vi "OpenAllNodes.vi"(0 "Task":T1(ring)) -> (2 "Nodes":cluster{"node":string, "Node Port":i32}[](array[cluster]))   [LabVIEW 2012]
uses:
  SubVIs/_ROSControl.ctl
  SubVIs/_ROSDirection.ctl
  _ROSDefinition.vi
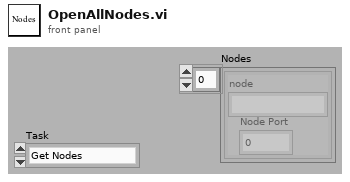
[diagram p1: front panel]
types:
  T1 = enum16{"Get Nodes", "Start Nodes", "Reset Nodes"}
  T2 = typedef "_ROSControl.ctl" = cluster{"topic port":u16, "Node":string, "topic":string, "type":string, "node port":u32, "error ":errorcluster, "Direction":T3, "APIs":string[], "Update (ms)":u16, "write queue":u16}
  T3 = typedef "_ROSDirection.ctl" = enum16{"Node", "Publisher", "Subscriber", "Service Client"}
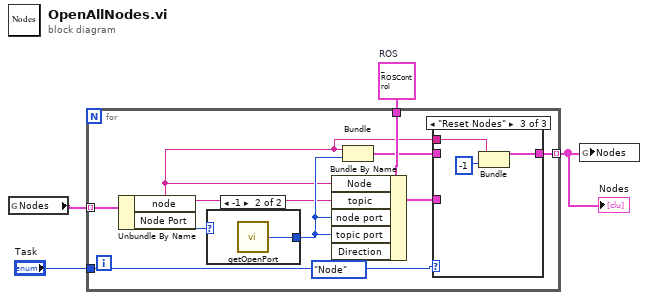
[diagram p0: block diagram]
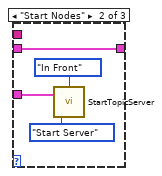
[diagram p3: hidden frame]
diagram:
  w4 = T2 {"topic port"=0, "Node"="", "topic"="", "type"="", "node port"=0, "error "={"status"=FALSE, "code"=0, "source"=""}, "Direction"=enum."Node", "APIs"=[], "Update (ms)"=0, "write queue"=0}  # ROS
  n1 = global read "_ROSDefinition.vi" "Nodes"() -> (w2:cluster{"node":string, "Node Port":i32}[])
  n2 = for {
    tunnel: w2 -> [w14] mode=indexing
    tunnel: w4 -> [w13]
    tunnel: [w6] -> w3 mode=indexing
    tunnel: "Task" -> [w8]
    n3 = Unbundle By Name(w14) -> ("node"=w7:string, "Node Port"=w10:i32)
    n4 = case shown="-1" w10 {
      selector: w10 -> [w23 _]
      tunnel: [w23 w24] -> w9
      frame Default {
      }
      frame -1 {
        n5 = call "getOpenPort.vi"() -> ("port"=w24:u16)
      }
    }
    n6 = Bundle By Name(cluster=w13, "Node"=w7, "topic"=w7, "node port"=w9, "topic port"=w9, "Direction"=_ROSDirection."Node") -> (w11:T2)
    n7 = Bundle("node"=w7, "Node Port"=w9) -> (w5:cluster{"node":string, "Node Port":i32})  [unwired: 1 in]
    n8 = case shown="\"Reset Nodes\"" w8 {
      tunnel: w11 -> [_ w19 _]
      tunnel: w7 -> [_ _ w22]
      tunnel: [w15 w16 w20] -> w6
      tunnel: w5 -> [w15 w16 _]
      frame "Get Nodes", Default {
      }
      frame "Start Nodes" {
        n9 = call "StartTopicServer.vi"("Server Direction"=enum16{"Start Server", "Close Server"}."Start Server", "ROS in"=w19, "Priority"=enum16{"In Front", "In Back"}."In Front") -> ()  [unwired: 1 in, 1 out]
      }
      frame "Reset Nodes" {
        n10 = Bundle("node"=w22, -1) -> (w20:cluster{"node":string, i32})  [unwired: 1 in]
      }
    }
  }
  "Nodes" <- w3
  n11 = global write "_ROSDefinition.vi" "Nodes"(w3) -> ()
